vi "SDO_SIM_SIM_MODULE_INIT.vi"(3 "Module Index":i32, 4 "SwerveRadiansPerCount":dbl=1.0, 5 "Drive PWM Channel":T2, 6 "DriveDistPerCount":dbl=1.0, 7 "Swerve PWM Channel":T2, 8 "Swerve B Channel":T1, 9 "Swerver A Channel":T1, 10 "Drive B Channel":T1, 11 "Drive A channel":T1) -> ()   [LabVIEW 2019]
uses:
  <vilib>/Rock Robotics/SystemInterfaces/DIO/FPGA_DIOChannel.ctl
  <vilib>/Rock Robotics/SystemInterfaces/DIO/FPGA_DIOPWMChannel.ctl
  SDO_SIM_SIM_Globals.vi
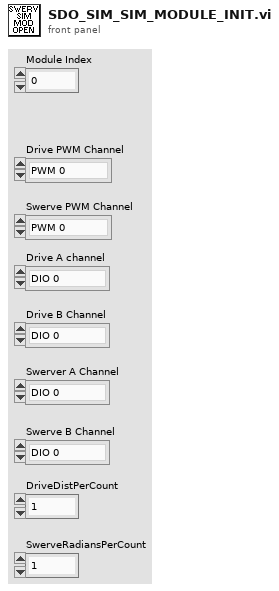
[diagram p1: front panel]
types:
  T1 = typedef "FPGA_DIOChannel.ctl" = enum8{"DIO 0", "DIO 1", "DIO 2", "DIO 3", "DIO 4", "DIO 5", "DIO 6", "DIO 7", "DIO 8", "DIO 9", "DIO MXP 0", "DIO MXP 1", "DIO MXP 2", "DIO MXP 3", "DIO MXP 4", "DIO MXP 5", "DIO MXP 6", "DIO MXP 7", "DIO MXP 8", "DIO MXP 9", "DIO MXP 10", "DIO MXP 11", "DIO MXP 12", "DIO MXP 13", "DIO MXP 14", "DIO MXP 15", "SPI Port CS1", "SPI Port CS2", "SPI Port CS3", "SPI Port MISO", "SPI Port MOSI", "Invalid"}
  T2 = typedef "FPGA_DIOPWMChannel.ctl" = enum8{"PWM 0", "PWM 1", "PWM 2", "PWM 3", "PWM 4", "PWM 5", "PWM 6", "PWM 7", "PWM 8", "PWM 9", "PWM MXP 0", "PWM MXP 1", "PWM MXP 2", "PWM MXP 3", "PWM MXP 4", "PWM MXP 5", "PWM MXP 6", "PWM MXP 7", "PWM MXP 8", "PWM MXP 9", "Invalid"}
  T3 = cluster{"Swerve Motor Device Index":i32, "Drive Motor Device Index":i32, "Swerve Encoder Device Index":i32, "Drive Encoder Device Index":i32, "Drive DistPerzcount":dbl, "SwerveRadPerCount":dbl}[]
  T4 = typedef "SDO_DRIVE_MODULE_TYPDEF.ctl" = cluster{"SwervDriveMotor":T5, "SwerveSwerveMotor":T5, "SwerveDriveEnc":T8, "SwerveSwerveEnc":T8}
  T5 = typedef "WPI_MotorControlDeviceRef.ctl" = cluster{"DeviceStatus":errorcluster, "Type":T6, "PWM":cluster{"PWM Channel":T2, "DeadBand":T7}, "CAN":cluster{"Device Number":u8, "SetOutput VI Ref":variant, "GetOutput VI Ref":variant, "Enable VI Ref":variant, "Disable VI Ref":variant, "Data":variant}, "Invert":bool, "DIO PWM":cluster{"PWM \"Enable\" Channel":T2, "DIOChannel":T1, "PWM Rate":dbl}}
  T6 = typedef "WPI_MotorControlType.ctl" = enum16{"PWM", "CAN", "DIO PWM"}
  T7 = typedef "WPI_PWMDeadband.ctl" = cluster{"Name":string, "maxPositivePwm":i32, "minPositivePwm":i32, "centerPwm":i32, "maxNegativePwm":i32, "minNegativePwm":i32, "angularRange":u16}
  T8 = typedef "WPI_EncoderDevRef.ctl" = cluster{"DevStatus":errorcluster, "EncoderIndex":T9, "CounterIndex":T10, "DistancePerCount":dbl, "Decoding Type":T11}
  T9 = typedef "FPGA_EncoderIdx.ctl" = enum8{"Enc 0", "Enc 1", "Enc 2", "Enc 3", "Enc 4", "Enc 5", "Enc 6", "Enc 7", "Invalid"}
  T10 = typedef "FPGA_CounterCtrSystemIndex.ctl" = enum8{"Ctr 0", "Ctr 1", "Ctr 2", "Ctr 3", "Ctr 4", "Ctr 5", "Ctr 6", "Ctr 7", "Invalid"}
  T11 = typedef "WPI_EncoderType.ctl" = enum16{"1x", "2x", "4x"}
  T12 = cluster{"Swerve Motor Device Index":i32, "Drive Motor Device Index":i32, "Swerve Encoder Device Index":i32, "Drive Encoder Device Index":i32, "Drive DistPerzcount":dbl, "SwerveRadPerCount":dbl}
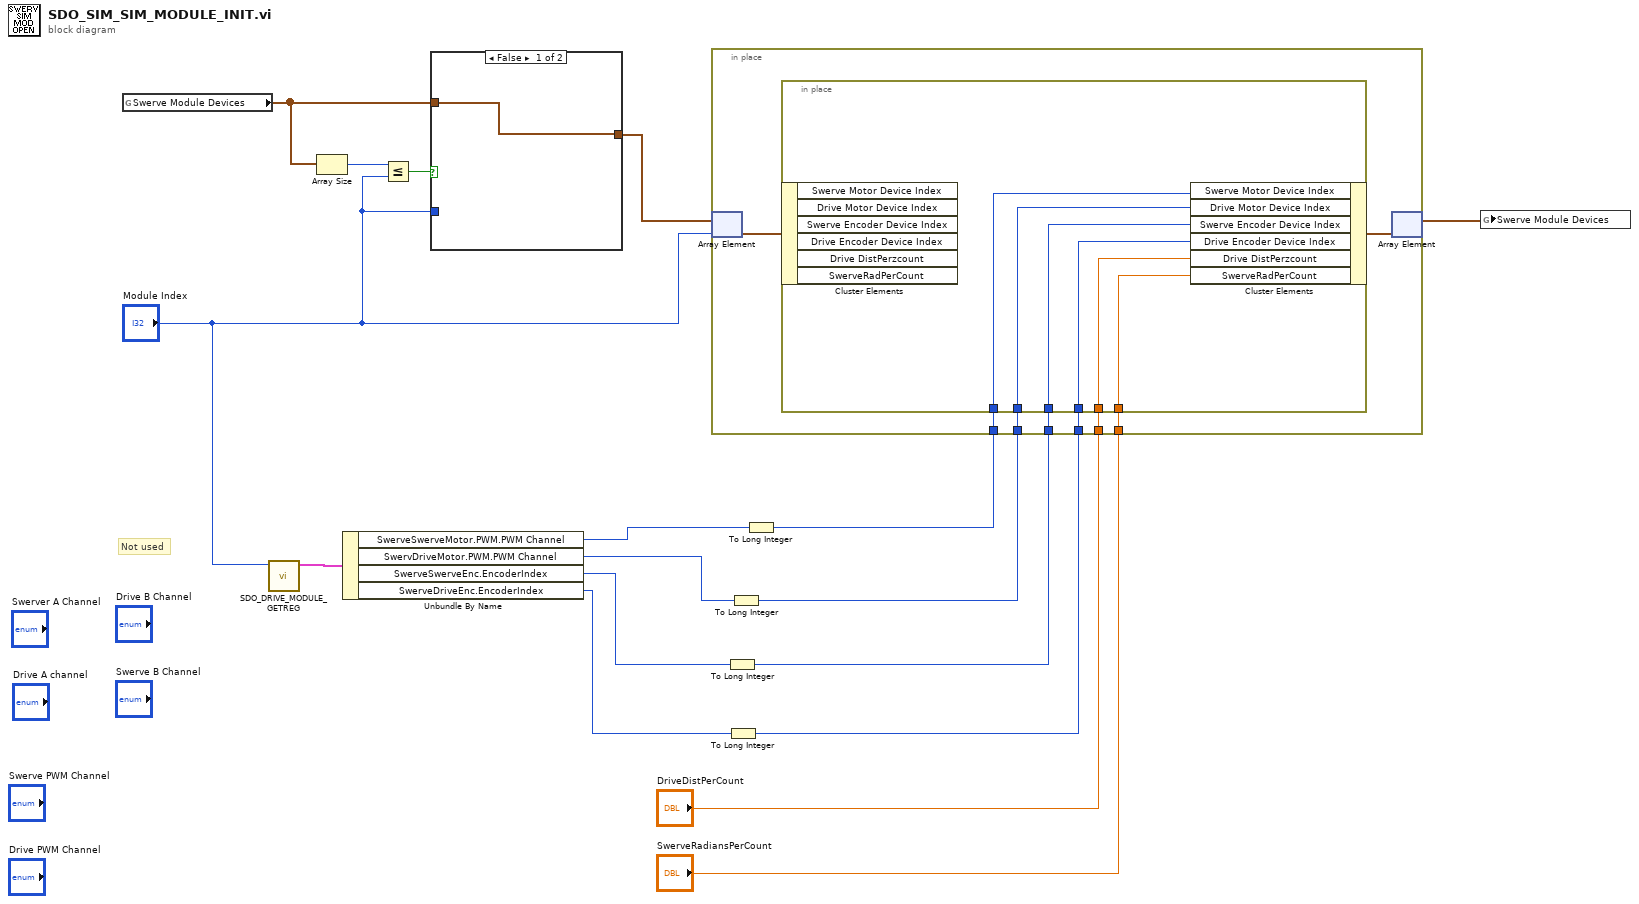
[diagram p0: block diagram]
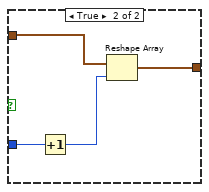
[diagram p2: hidden frame]
diagram:
  # "Not used"
  n1 = global read "SDO_SIM_SIM_Globals.vi" "Swerve Module Devices"() -> (w8:T3)
  n2 = call "SDO_DRIVE_MODULE_GETREG.vi"("Suffix"="Module Index") -> ("Swerve Module TypDef"=w6:T4)  [unwired: 10 in]
  n3 = Array Size(array=w8) -> (size(s)=w10:i32)
  n4 = Unbundle By Name(w6) -> ("SwerveSwerveMotor.PWM.PWM Channel"=w2:T2, "SwervDriveMotor.PWM.PWM Channel"=w1:T2, "SwerveSwerveEnc.EncoderIndex"=w4:T9, "SwerveDriveEnc.EncoderIndex"=w3:T9)
  n5 = Less Or Equal?(x=w10, y="Module Index") -> (x <= y?=w9:bool)
  n6 = case shown="False" w9 {
    tunnel: w8 -> [w18 w20]
    tunnel: "Module Index" -> [_ w22]
    tunnel: [w18 w19] -> w7
    frame False {
    }
    frame True {
      n7 = Increment(x=w22) -> (x+1=w21:i32)
      n8 = Reshape Array(w20, w21) -> (w19:T3)
    }
  }
  n9 = To Long Integer(number=w4) -> (32bit integer=w14:i32)
  n10 = To Long Integer(number=w3) -> (32bit integer=w13:i32)
  n11 = To Long Integer(number=w1) -> (32bit integer=w15:i32)
  n12 = To Long Integer(number=w2) -> (32bit integer=w16:i32)
  n13 = in-place {
    in-place-border: w16 -> [w29]
    in-place-border: w15 -> [w28]
    in-place-border: w14 -> [w26]
    in-place-border: w13 -> [w25]
    in-place-border: "DriveDistPerCount" -> [w24]
    in-place-border: "SwerveRadiansPerCount" -> [w23]
    n14 = in-place-array #1(w7, "Module Index") -> (w30:T12)
    n15 = in-place {
      in-place-border: w29 -> [w36]
      in-place-border: w28 -> [w35]
      in-place-border: w26 -> [w34]
      in-place-border: w25 -> [w33]
      in-place-border: w24 -> [w32]
      in-place-border: w23 -> [w31]
      n16 = in-place-cluster #2(w30) -> ()  [unwired: 6 out]
      n17 = in-place-cluster #2("Swerve Motor Device Index"=w36, "Drive Motor Device Index"=w35, "Swerve Encoder Device Index"=w34, "Drive Encoder Device Index"=w33, "Drive DistPerzcount"=w32, "SwerveRadPerCount"=w31) -> (w27:T12)
    }
    n18 = in-place-array #1(w27) -> (w17:T3)  [unwired: 1 out]
  }
  n19 = global write "SDO_SIM_SIM_Globals.vi" "Swerve Module Devices"(w17) -> ()
